vi "Example XYGraph Markers - 副本.vi"() -> ()   [LabVIEW 2020]
doc: "Graph extensions add the ability to have very capable and interactive markers placed on the graph. This GRAPH control has a custom palette icon for the \"cursor\" mode, which is replaced by graph extensions' markers mode.\n\nThis markers extension, has by default the the cursors extension included, which is activated automatically in the various other graph palette active tools. (like pan, zoom)."
uses:
  controls/commands.ctl
  <vilib>/ptbypt/NI_PtbyPt.lvlib
  Graph Extensions.lvlib
panel:
  out "XY Graph":cluster{dbl[], dbl[]}[](graph)
  # "Instructions:\n1. Run the VI, move the mouse over the graph.  \n2. The graph has to be in cursor (marker)mode to enable markers (the right hand button)\n3. Left click to follow instructions and place markers\n4. Right click to change the marker type, options or edit existing markers.\n5. Switch graph tools, to pan and markers will follow automatically."
  # "The cursor icon has been replaced for use\nwith the markers in graph extensions"
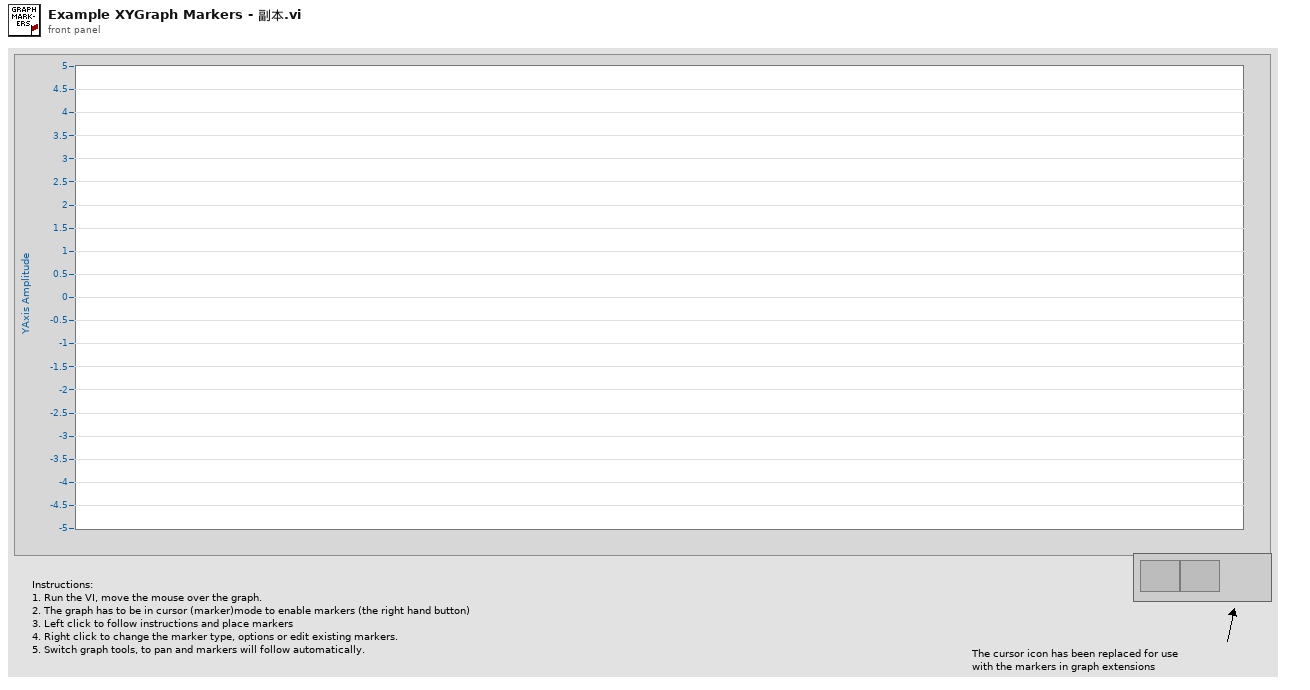
[diagram p1: front panel]
types:
  T1 = typedef "Graph Extensions.lvlib/commands.ctl" = enum16{"up", "options", "click", "move", "type", "redraw", "edited", "exit", "Mark"}
  T2 = typedef "LVPoint32TypeDef.ctl" = cluster{"Horizontal":i32, "Vertical":i32}
  T3 = typedef "Graph Extensions.lvlib/markerType.ctl" = enum16{"point", "arrow", "horiz", "vert", "vert range", "horiz range", "box"}
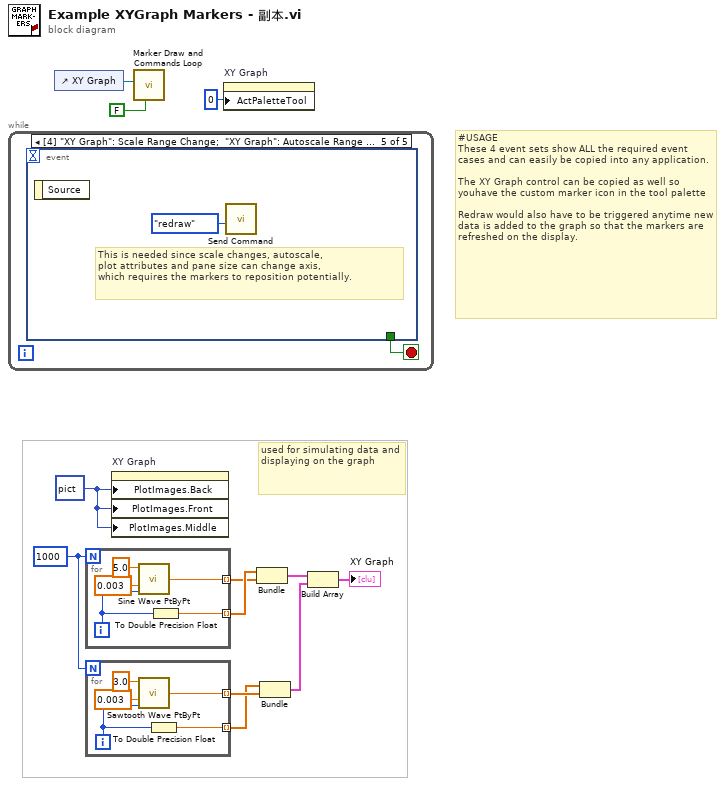
[diagram p0: block diagram]
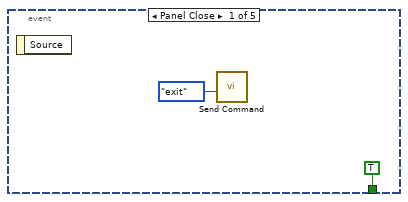
[diagram p2: hidden frame]
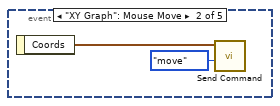
[diagram p3: hidden frame]
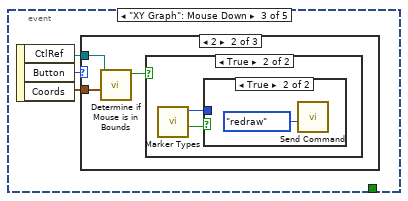
[diagram p4: hidden frame]
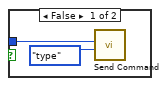
[diagram p7: hidden frame]
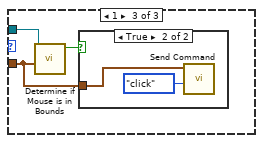
[diagram p8: hidden frame]
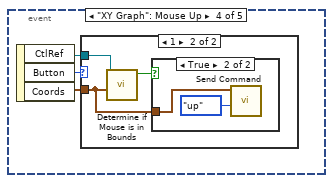
[diagram p10: hidden frame]
diagram:
  w4 = picture data[5B] ("Plot Images:Back")
  w5 = 1000
  # "#USAGE\nThese 4 event sets show ALL the required event cases and can easily be copied into any application.\n\nThe XY Graph control can be copied as well so youhave the custom marker icon in the tool palette\n\nRedraw would also have to be triggered anytime new data is added to the graph so that the markers are refreshed on the display."
  # "used for simulating data and displaying on the graph"
  n1 = while {
    stop <- w13 stop-if-true
    n2 = event shown="[4] \"XY Graph\": Scale Range Change;  \"XY Graph\": Autoscale Range Change;  \"XY Graph\": Plot Attribute Change;  \"Pane\": Pane Size" {
      selector: _ -> [_ _ _ _ _]
      dyn-events: _ -> [_ _ _ _ _]
      timeout: _ -> [_ _ _ _ _]
      tunnel: [TRUE _ _ _ _] -> w13
      event Panel Close {
        n3 = event-data() -> ()  [unwired: 1 in, 1 out]
        n4 = call "Send Command.vi"("cmd"=commands."exit") -> ()  [unwired: 11 in]
      }
      event "XY Graph": Mouse Move {
        n5 = event-data() -> ("Coords"=w17:T2)  [unwired: 1 in]
        n6 = call "Send Command.vi"("cmd"=commands."move", "Coords"=w17) -> ()  [unwired: 10 in]
      }
      event "XY Graph": Mouse Down {
        n7 = event-data() -> ("CtlRef"=w18:refnum<vi>, "Button"=w20:u16, "Coords"=w19:T2)  [unwired: 1 in]
        n8 = case shown="2" w20 {
          tunnel: w19 -> [_ w23 w30]
          tunnel: w18 -> [_ w22 w31]
          frame Default {
          }
          frame 2 {
            n9 = call "Determine if Mouse is in Bounds.vi"("Coords"=w23, "XYGraph in"=w22) -> ("In bounds?"=w21:bool)  [unwired: 9 in]
            n10 = case shown="True" w21 {
              frame False {
              }
              frame True {
                n11 = call "Marker Types.vi"() -> ("Close"=w25:bool, "Type"=w24:T3)  [unwired: 10 in]
                n12 = case shown="True" w25 {
                  tunnel: w24 -> [w27 _]
                  frame False {
                    n13 = call "Send Command.vi"("cmd"=commands."type", "Type"=w27) -> ()  [unwired: 10 in]
                  }
                  frame True {
                    n14 = call "Send Command.vi"("cmd"=commands."redraw") -> ()  [unwired: 11 in]
                  }
                }
              }
            }
          }
          frame 1 {
            n15 = call "Determine if Mouse is in Bounds.vi"("Coords"=w30, "XYGraph in"=w31) -> ("In bounds?"=w29:bool)  [unwired: 9 in]
            n16 = case shown="True" w29 {
              tunnel: w30 -> [_ w32]
              frame False {
              }
              frame True {
                n17 = call "Send Command.vi"("cmd"=commands."click", "Coords"=w32) -> ()  [unwired: 10 in]
              }
            }
          }
        }
      }
      event "XY Graph": Mouse Up {
        n18 = event-data() -> ("CtlRef"=w34:refnum<vi>, "Button"=w36:u16, "Coords"=w35:T2)  [unwired: 1 in]
        n19 = case shown="1" w36 {
          tunnel: w35 -> [_ w38]
          tunnel: w34 -> [_ w39]
          frame Default {
          }
          frame 1 {
            n20 = call "Determine if Mouse is in Bounds.vi"("Coords"=w38, "XYGraph in"=w39) -> ("In bounds?"=w37:bool)  [unwired: 9 in]
            n21 = case shown="True" w37 {
              tunnel: w38 -> [_ w40]
              frame False {
              }
              frame True {
                n22 = call "Send Command.vi"("cmd"=commands."up", "Coords"=w40) -> ()  [unwired: 10 in]
              }
            }
          }
        }
      }
      event "XY Graph": Scale Range Change; "XY Graph": Autoscale Range Change; "XY Graph": Plot Attribute Change; Pane Size {
        # "This is needed since scale changes, autoscale, \nplot attributes and pane size can change axis, \nwhich requires the markers to reposition potentially."
        n23 = event-data() -> ()  [unwired: 1 in, 1 out]
        n24 = call "Send Command.vi"("cmd"=commands."redraw") -> ()  [unwired: 11 in]
      }
    }
  }
  n25 = control-ref of="XY Graph"() -> (w2:refnum<vi>)
  n26 = for {
    N: w5 -> [_]
    tunnel: [w47] -> w11 mode=indexing
    tunnel: [w43] -> w12 mode=indexing
    i -> [w46]
    n27 = call <vilib>:"Sine Wave PtByPt.vi"("time"=w46, "frequency"=0.003, "amplitude"=5.0) -> ("sine wave"=w47:dbl)  [unwired: 1 in]
    n28 = To Double Precision Float(number=w46) -> (double precision float=w43:dbl)
  }
  n29 = for {
    N: w5 -> [_]
    tunnel: [w52] -> w8 mode=indexing
    tunnel: [w48] -> w7 mode=indexing
    i -> [w51]
    n30 = call <vilib>:"Sawtooth Wave PtByPt.vi"("time"=w51, "frequency"=0.003, "amplitude"=3.0) -> ("sawtooth wave"=w52:dbl)  [unwired: 1 in]
    n31 = To Double Precision Float(number=w51) -> (double precision float=w48:dbl)
  }
  n32 = property on="XY Graph" class="XYGraph (strict)"("PlotImages.Back"=w4, "PlotImages.Front"=w4, "PlotImages.Middle"=w4) -> ()  [unwired: 2 in, 2 out]
  n33 = call "Marker Draw and Commands Loop.vi"("Enable Cursors"=FALSE, "XY Graph"=w2) -> ()  [unwired: 10 in]
  n34 = property on="XY Graph" class="XYGraph (strict)"("ActPaletteTool"=0 ("Palette:Active Tool")) -> ()  [unwired: 2 in, 2 out]
  n35 = Bundle(w12, w11) -> (w10:cluster{dbl[], dbl[]})  [unwired: 1 in]
  n36 = Bundle(w7, w8) -> (w6:cluster{dbl[], dbl[]})  [unwired: 1 in]
  n37 = Build Array(w10, w6) -> (→"XY Graph":cluster{dbl[], dbl[]}[])
